vi "OTP - Main UI.vi"() -> ()   [LabVIEW 2020]
uses:
  Tab control.ctl
panel:
  in  "Back":bool
  in  "Tab Control":T1=enum."Source data"
  in  "Equipment":enum16{"VNA", "LCR"}(ring) caption="Equipment used for the beam data"
  in  "Measurement file (csv)":path
  in  "Frequency (MHz)":dbl=837.0
  in  "Package number":string="08"
  out "Cmax (fF)":dbl caption="Cmax measured (fF)"
  out "Cmin (fF)":dbl caption="Cmin measured (fF)"
  in  "Specification":T2={"Cmin (fF)"=500.0, "Cmin tolerance (%)"=10.0, "Cmax (fF)"=3460.0, "Cmax tolerance (%)"=1.38, "States"=32}
  out "Register 2 & 3 (hex) 2":string[][](array[string]) caption="Registers 2 & 3 (hex) to be considered"
  out "Register 2 & 3 (hex)":u8[][](array[numeric]) caption="Proposal for programming Register 2 & 3 (dec)"
  out "Results":dbl[][](array[numeric]) caption="Spec, Emulated, Error"
  in  "Save header":bool=TRUE
  in  "Write to device":bool=TRUE
  in  "Delay":u32=200 caption="Delay between writes (ms)"
  in  "PIC COM-port":refnum<visa-resource-name>
  in  "DUT info to write":T3={"Serial Number"=11, "Specification ID"="1A", "Variant"="W0", "Package"="22"}
  out "Status":string
  in  "Stop":bool
  in  "Forward":bool
  out "error out":errorcluster
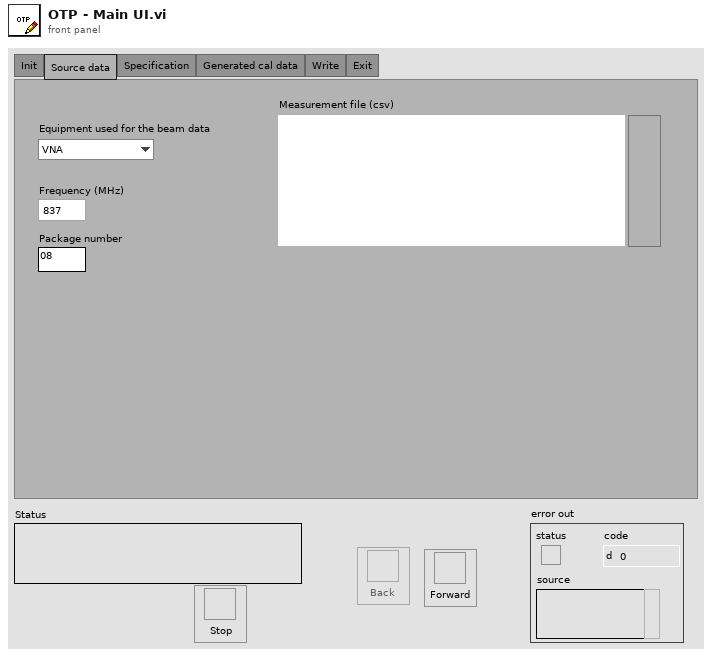
[diagram p1: front panel]
types:
  T1 = typedef "Tab control.ctl" = enum32{"Init", "Source data", "Specification", "Generated cal data", "Write", "Exit"}
  T2 = cluster{"Cmin (fF)":dbl, "Cmin tolerance (%)":dbl, "Cmax (fF)":dbl, "Cmax tolerance (%)":dbl, "States":i32}
  T3 = cluster{"Serial Number":u16, "Specification ID":string, "Variant":string, "Package":string}
  T4 = cluster{"Specification":cluster{"Cmin (fF)":dbl, "Cmin tolerance (%)":dbl, "Cmax (fF)":dbl, "Cmax tolerance (%)":dbl, "States":i32}, "Register 2 & 3 (hex)":string[][], "dCap (fF)":dbl[], "Cmin (fF)":dbl, "Cmax (fF)":dbl}
  T5 = cluster{"Package number":string, "Frequency (MHz)":dbl, "Measurement file (csv)":path, "Equipment":enum16{"VNA", "LCR"}}
  T6 = enum8{"Enabled", "Disabled", "Disabled and Grayed Out"}
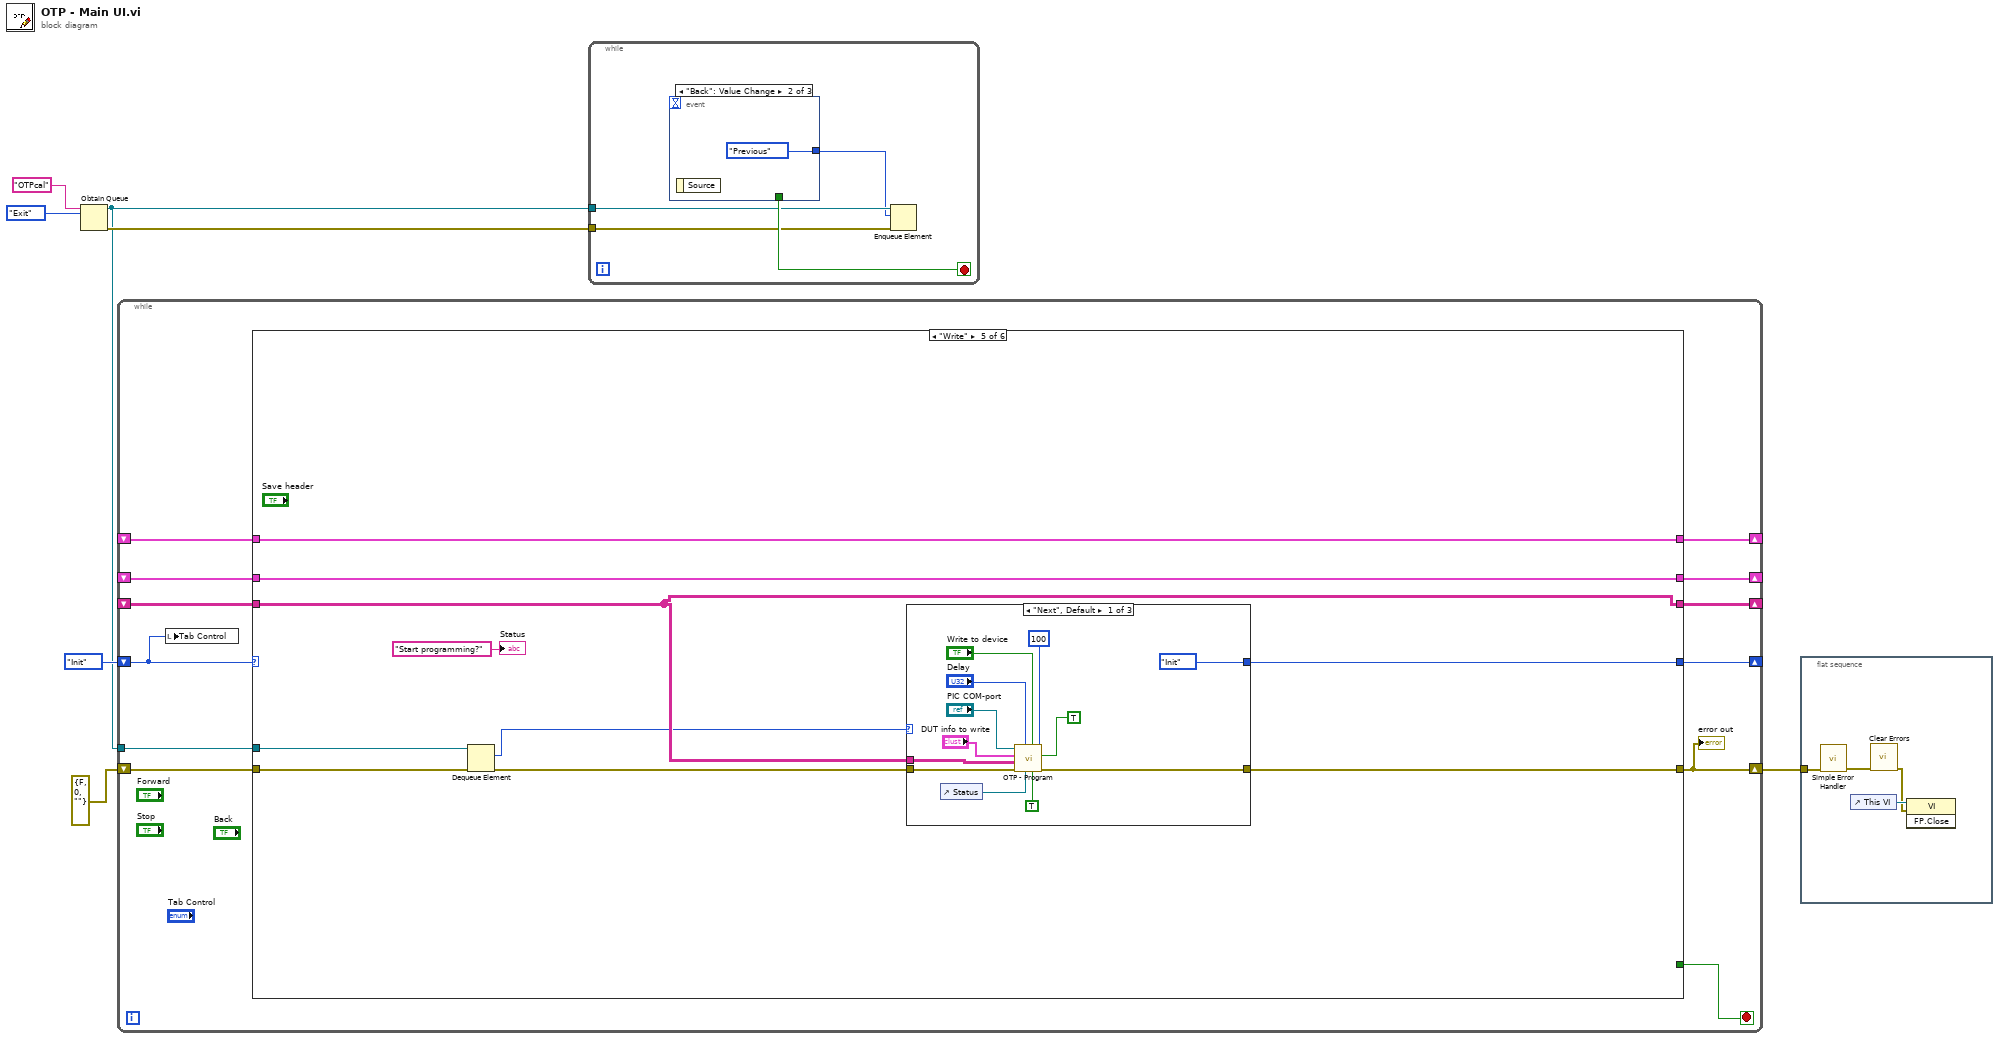
[diagram p0: block diagram]
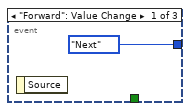
[diagram p2: hidden frame]
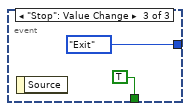
[diagram p3: hidden frame]
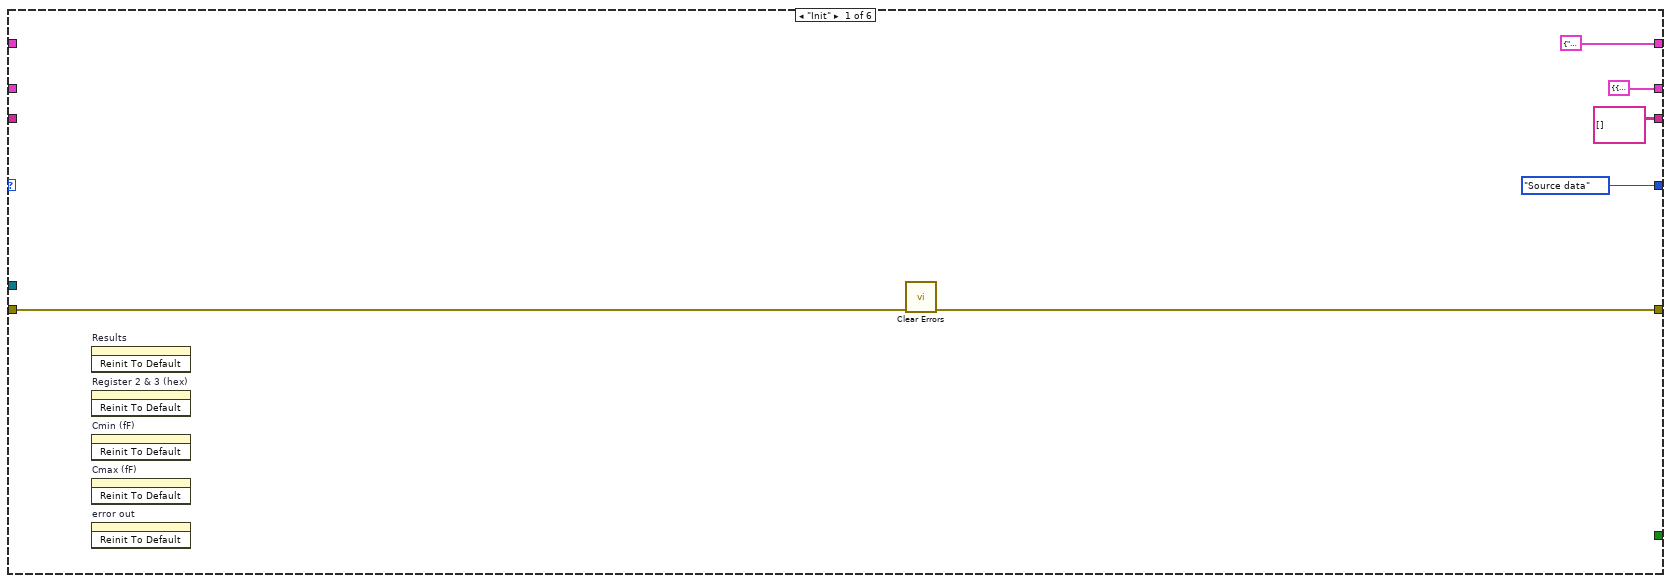
[diagram p4: hidden frame]
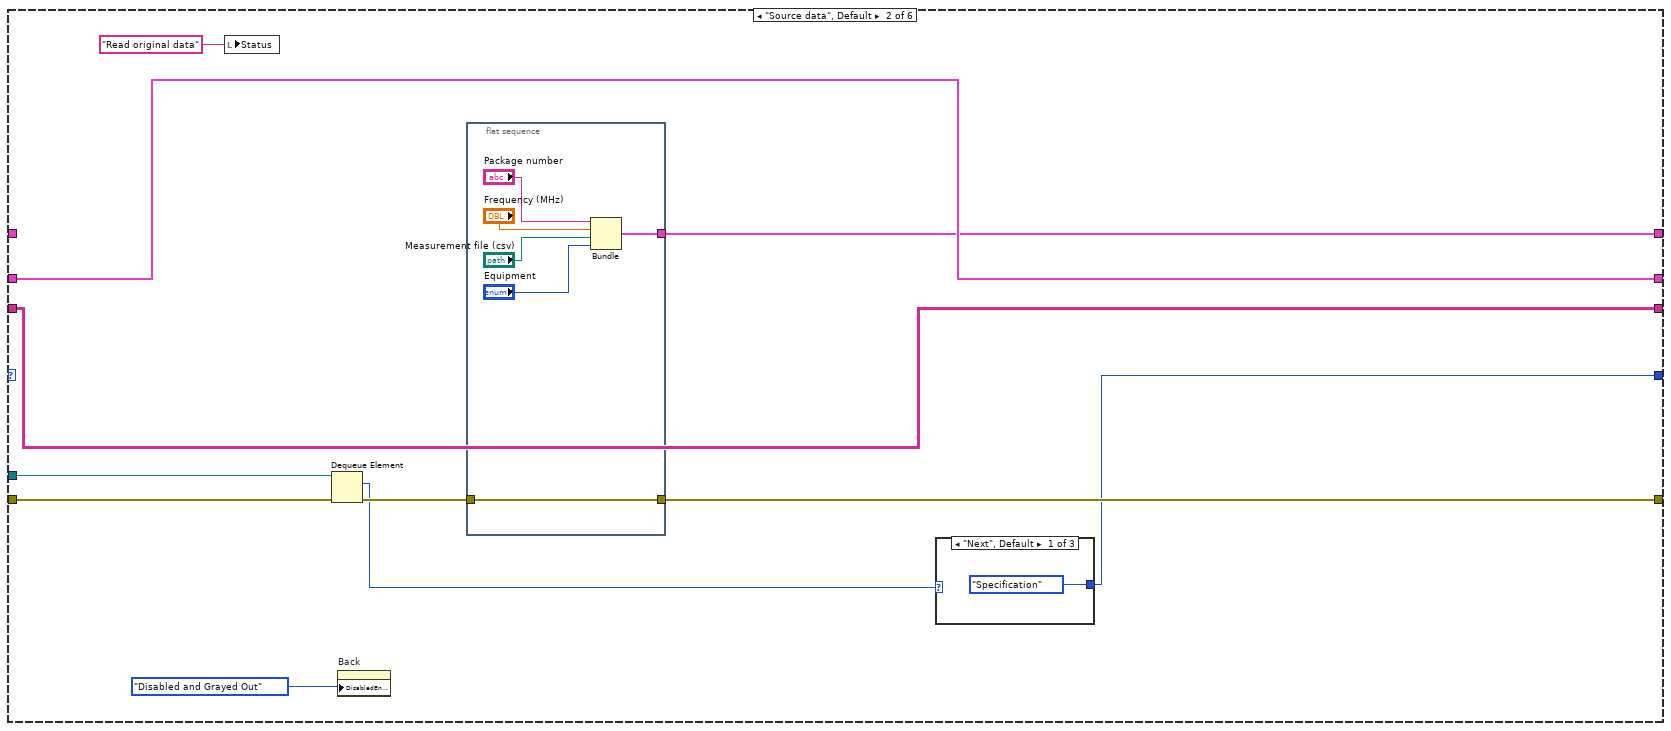
[diagram p5: hidden frame]
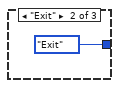
[diagram p6: hidden frame]
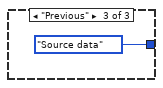
[diagram p7: hidden frame]
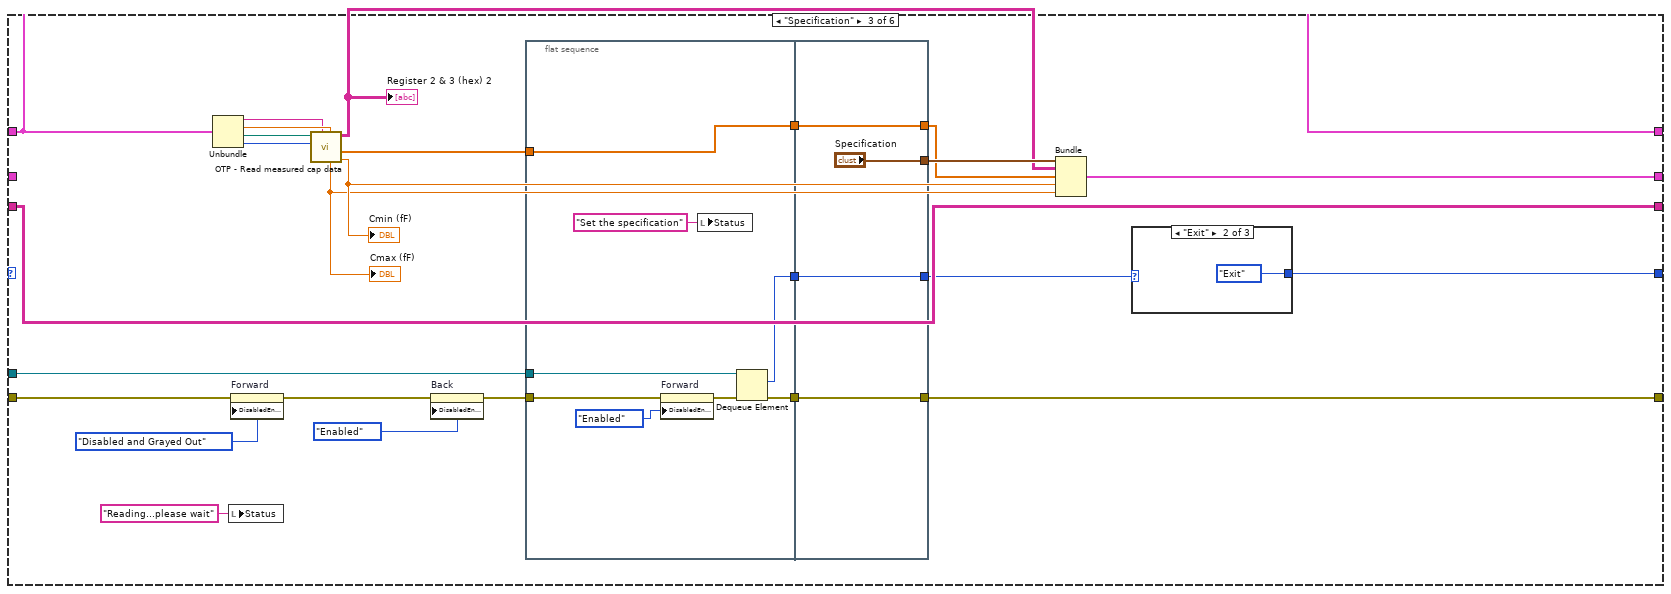
[diagram p8: hidden frame]
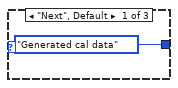
[diagram p9: hidden frame]
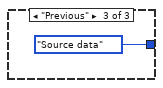
[diagram p10: hidden frame]
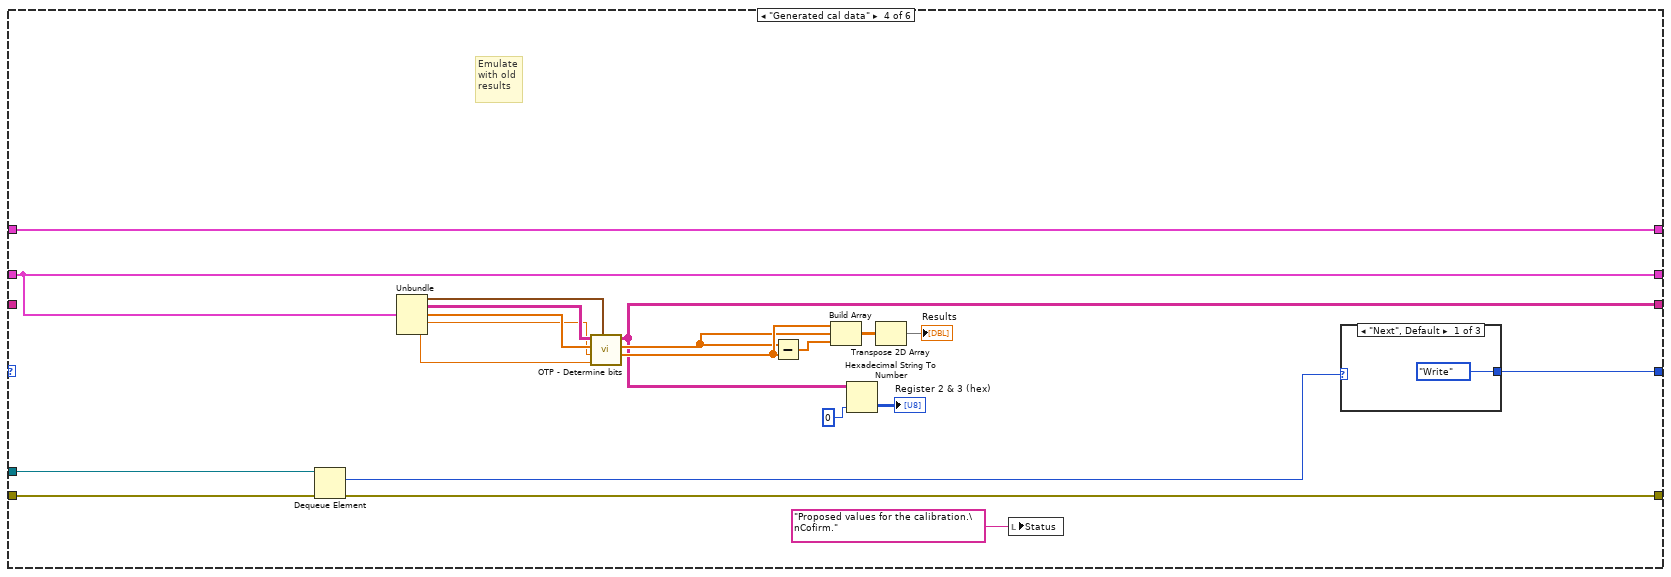
[diagram p11: hidden frame]
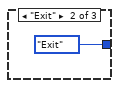
[diagram p12: hidden frame]
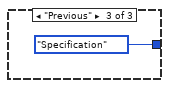
[diagram p13: hidden frame]
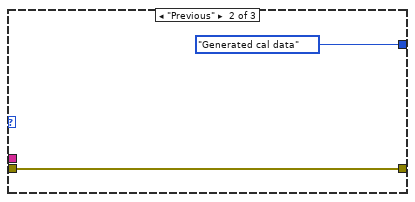
[diagram p14: hidden frame]
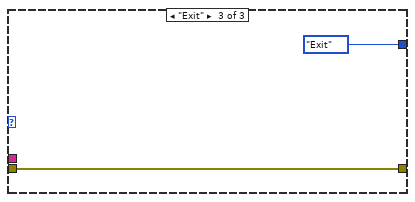
[diagram p15: hidden frame]
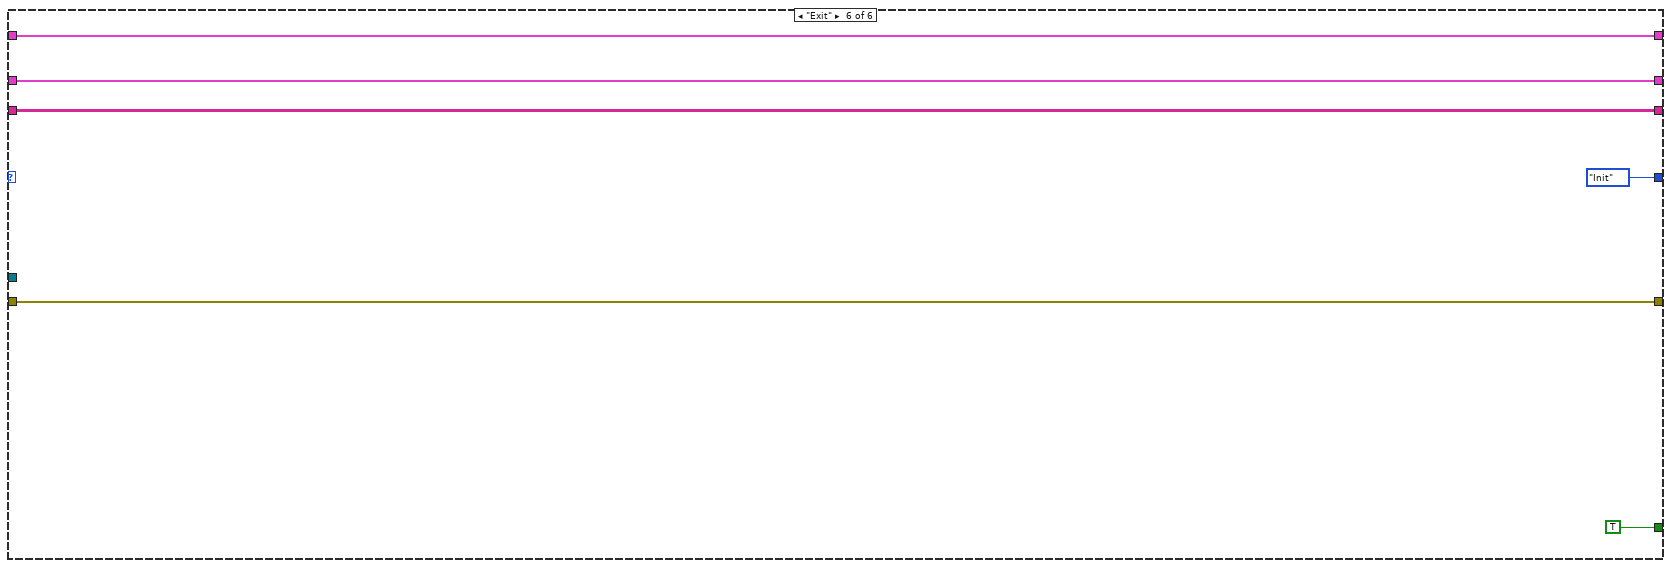
[diagram p16: hidden frame]
diagram:
  n1 = Obtain Queue(name (unnamed)="OTPcal", element data type=enum16{"Next", "Previous", "Exit"}."Exit") -> (queue out=w1:refnum<queue>, error out=w2:errorcluster)  [unwired: 3 in, 1 out]
  n2 = while {
    shift-right: [w18] -> _
    shift-left: Tab_control."Init" ("Tab Control") -> [w19]
    shift-right: [w10] -> _
    shift-left: _ -> [w16]
    shift-right: [w17] -> _
    shift-left: _ -> [w15]
    shift-right: [w14] -> _
    shift-left: _ -> [w13]
    shift-right: [w9] -> w6
    shift-left: errorcluster {"status"=FALSE, "code"=0, "source"=""} ("error out 2") -> [w12]
    tunnel: w1 -> [w8]
    stop <- w11 stop-if-true
    n3 = local write "Tab Control"(w19) -> ()
    n4 = case shown="\"Write\"" w19 {
      tunnel: [Tab_control."Source data" ("Tab Control") w27 w46 w88 w111 Tab_control."Init" ("Tab Control")] -> w18
      tunnel: [T5 {"Package number"="", "Frequency (MHz)"=0.0, "Measurement file (csv)"=path "", "Equipment"=enum."VNA"} w34 w56 w95 w117 w140] -> w10
      tunnel: [T4 {"Specification"={"Cmin (fF)"=0.0, "Cmin tolerance (%)"=0.0, "Cmax (fF)"=0.0, "Cmax tolerance (%)"=0.0, "States"=0}, "Register 2 & 3 (hex)"=[], "dCap (fF)"=[], "Cmin (fF)"=0.0, "Cmax (fF)"=0.0} w36 w61 w94 w118 w141] -> w17
      tunnel: w16 -> [_ _ w56 w95 w117 w140]
      tunnel: w15 -> [_ w36 _ w94 w118 w141]
      tunnel: [string[][] [] ("Register 2 & 3 (hex)") w35 w57 w96 w119 w142] -> w14
      tunnel: [w20 w30 w49 w90 w120 w138] -> w9
      tunnel: w13 -> [_ w35 w57 _ w119 w142]
      tunnel: w12 -> [w21 w32 w59 w91 w113 w138]
      tunnel: [_ _ _ _ _ TRUE] -> w11
      tunnel: w8 -> [_ w29 w50 w89 w115 _]
      frame "Init" {
        n5 = invoke on="Results" class="Arr (strict)" method="Reinit To Default"() -> ()  [unwired: 3 in, 3 out]
        n6 = invoke on="Register 2 & 3 (hex)" class="Arr (strict)" method="Reinit To Default"() -> ()  [unwired: 3 in, 3 out]
        n7 = invoke on="Cmin (fF)" class="DigNum (strict)" method="Reinit To Default"() -> ()  [unwired: 3 in, 3 out]
        n8 = invoke on="Cmax (fF)" class="DigNum (strict)" method="Reinit To Default"() -> ()  [unwired: 3 in, 3 out]
        n9 = invoke on="error out" class="Clust (strict)" method="Reinit To Default"() -> ()  [unwired: 3 in, 3 out]
        n10 = call <vilib>:"Clear Errors.vi"("error in (no error)"=w21) -> ("error out"=w20:errorcluster)  [unwired: 5 in, 1 out]
      }
      frame "Source data", Default {
        n11 = local write "Status"("Read original data" ("String")) -> ()
        n12 = Dequeue Element(queue=w29, error in (no error)=w32) -> (element=w28:enum16{"Next", "Previous", "Exit"}, error out=w31:errorcluster)  [unwired: 1 in, 2 out]
        n13 = property on="Back" class="Bool"("DisabledEnum"=T6."Disabled and Grayed Out" ("Disabled")) -> ()  [unwired: 2 in, 2 out]
        n14 = flat-sequence {
          tunnel: [w45] -> w34
          tunnel: [w40] -> w30
          tunnel: w31 -> [w40]
          frame #0 {
            n15 = Bundle("Package number"="Package number", "Frequency (MHz)"="Frequency (MHz)", "Measurement file (csv)"="Measurement file (csv)", "Equipment"="Equipment") -> (w45:T5)  [unwired: 1 in]
          }
        }
        n16 = case shown="\"Next\", Default" w28 {
          tunnel: [Tab_control."Specification" ("Tab Control") Tab_control."Exit" ("Tab Control") Tab_control."Source data" ("Tab Control")] -> w27
          frame "Next", Default {
          }
          frame "Exit" {
          }
          frame "Previous" {
          }
        }
      }
      frame "Specification" {
        n17 = Unbundle(w56) -> ("Package number"=w64:string, "Frequency (MHz)"=w65:dbl, "Measurement file (csv)"=w66:path, "Equipment"=w67:enum16{"VNA", "LCR"})
        n18 = local write "Status"("Reading...please wait" ("String")) -> ()
        n19 = property on="Forward" class="Bool"(error in=w59, "DisabledEnum"=T6."Disabled and Grayed Out" ("Disabled")) -> (error out=w58:errorcluster)  [unwired: 1 in, 1 out]
        n20 = call "OTP - Read measured cap data.vi"("Frequency (MHz)"=w65, "Package number"=w64, "Equipment"=w67, "file (use dialog)"=w66) -> ("Cmin (fF)"=w71:dbl, "dCap (fF)"=w53:dbl[], "Register 2 & 3 (hex)"=w68:string[][], "Cmax (fF)"=w69:dbl)  [unwired: 3 in, 1 out]
        "Cmin (fF)" <- w71
        "Cmax (fF)" <- w69
        "Register 2 & 3 (hex) 2" <- w68
        n21 = property on="Back" class="Bool"(error in=w58, "DisabledEnum"=T6."Enabled" ("Disabled")) -> (error out=w51:errorcluster)  [unwired: 1 in, 1 out]
        n22 = flat-sequence {
          tunnel: [w77] -> w55
          tunnel: [w80] -> w54
          tunnel: w53 -> [w80]
          tunnel: w51 -> [w79]
          tunnel: w50 -> [w78]
          tunnel: [w76] -> w48
          tunnel: [w86] -> w47
          tunnel: ["Specification"] -> w70
          tunnel: w55 -> [w86]
          tunnel: [w84] -> w52
          tunnel: w54 -> [w84]
          tunnel: [w83] -> w49
          tunnel: w48 -> [w83]
          frame #0 {
            n23 = property on="Forward" class="Bool"(error in=w79, "DisabledEnum"=T6."Enabled" ("Disabled")) -> (error out=w82:errorcluster)  [unwired: 1 in, 1 out]
            n24 = local write "Status"("Set the specification" ("String")) -> ()
            n25 = Dequeue Element(queue=w78, error in (no error)=w82) -> (element=w77:enum16{"Next", "Previous", "Exit"}, error out=w76:errorcluster)  [unwired: 1 in, 2 out]
          }
          frame #1 {
          }
        }
        n26 = Bundle("Specification"=w70, "Register 2 & 3 (hex)"=w68, "dCap (fF)"=w52, "Cmin (fF)"=w71, "Cmax (fF)"=w69) -> (w61:T4)  [unwired: 1 in]
        n27 = case shown="\"Exit\"" w47 {
          tunnel: [Tab_control."Generated cal data" ("Tab Control") Tab_control."Exit" ("Tab Control") Tab_control."Source data" ("Tab Control")] -> w46
          frame "Next", Default {
          }
          frame "Exit" {
          }
          frame "Previous" {
          }
        }
      }
      frame "Generated cal data" {
        # "Emulate\nwith old\nresults"
        n28 = Dequeue Element(queue=w89, error in (no error)=w91) -> (element=w87:enum16{"Next", "Previous", "Exit"}, error out=w90:errorcluster)  [unwired: 1 in, 2 out]
        n29 = Unbundle(w94) -> ("Specification"=w101:T2, "Register 2 & 3 (hex)"=w100:string[][], "dCap (fF)"=w99:dbl[], "Cmin (fF)"=w98:dbl, "Cmax (fF)"=w97:dbl)
        n30 = call "OTP - Determine bits.vi"("Specification"=w101, "Cmax measured (fF)"=w97, "Cmin measured (fF)"=w98, "dCap (fF)"=w99, "Register 2 & 3 (hex)"=w100) -> ("Target values (fF)"=w103:dbl[], "Measured values (fF)"=w102:dbl[], "Register 2 & 3 (hex)"=w96:string[][])  [unwired: 4 in]
        n31 = Subtract(x=w102, y=w103) -> (x-y=w104:dbl[])
        n32 = Build Array(w103, w102, w104) -> (w107:dbl[][])
        n33 = Hexadecimal String To Number(string=w96, default (0uL)=u8 0 ("milliseconds to wait")) -> (number=→"Register 2 & 3 (hex)":u8[][])  [unwired: 1 in, 1 out]
        n34 = Transpose 2D Array(2D array=w107) -> (transposed array=→"Results":dbl[][])
        n35 = local write "Status"("Proposed values for the calibration.\nCofirm." ("String")) -> ()
        n36 = case shown="\"Next\", Default" w87 {
          tunnel: [Tab_control."Write" ("Tab Control") Tab_control."Exit" ("Tab Control") Tab_control."Specification" ("Tab Control")] -> w88
          frame "Next", Default {
          }
          frame "Exit" {
          }
          frame "Previous" {
          }
        }
      }
      frame "Write" {
        n37 = Dequeue Element(queue=w115, error in (no error)=w113) -> (element=w112:enum16{"Next", "Previous", "Exit"}, error out=w114:errorcluster)  [unwired: 1 in, 2 out]
        n38 = case shown="\"Next\", Default" w112 {
          tunnel: w119 -> [w132 _ _]
          tunnel: [w124 w133 w135] -> w120
          tunnel: w114 -> [w123 w133 w135]
          tunnel: [Tab_control."Init" ("Tab Control") Tab_control."Generated cal data" ("Tab Control") Tab_control."Exit" ("Tab Control")] -> w111
          frame "Next", Default {
            n39 = control-ref of="Status"() -> (w125:refnum<vi>)
            n40 = call "OTP - Program.vi"("Save header"=TRUE, "Max number of retries"=100, "Read back the values written"=TRUE, "Write to device"="Write to device", "Str Refnum"=w125, "Delay"="Delay", "Error In"=w123, "OTP-cal registers 2 & 3 (hex)"=w132, "DUT info to write"="DUT info to write", "VISA resource name"="PIC COM-port") -> ("error out"=w124:errorcluster)  [unwired: 1 in]
          }
          frame "Previous" {
          }
          frame "Exit" {
          }
        }
        "Status" <- "Start programming?" ("String")
      }
      frame "Exit" {
      }
    }
    "error out" <- w9
  }
  n41 = while {
    tunnel: w1 -> [w145]
    tunnel: w2 -> [w144]
    stop <- w146 stop-if-true
    n42 = event shown="[1] \"Back\": Value Change" {
      selector: _ -> [_ _ _]
      dyn-events: _ -> [_ _ _]
      timeout: _ -> [_ _ _]
      tunnel: [enum16{"Next", "Previous", "Exit"}."Next" enum16{"Next", "Previous", "Exit"}."Previous" enum16{"Next", "Previous", "Exit"}."Exit"] -> w143
      tunnel: [_ _ TRUE] -> w146
      event "Forward": Value Change {
        n43 = event-data() -> ()  [unwired: 1 in, 1 out]
      }
      event "Back": Value Change {
        n44 = event-data() -> ()  [unwired: 1 in, 1 out]
      }
      event "Stop": Value Change {
        n45 = event-data() -> ()  [unwired: 1 in, 1 out]
      }
    }
    n46 = Enqueue Element(queue=w145, element=w143, error in (no error)=w144) -> ()  [unwired: 1 in, 3 out]
  }
  n47 = flat-sequence {
    tunnel: w6 -> [w153]
    frame #0 {
      n48 = call <vilib>:"Simple Error Handler.vi"("error in (no error)"=w153) -> ("error out"=w152:errorcluster)  [unwired: 4 in, 4 out]
      n49 = control-ref of="This VI"() -> (w154:refnum<vi>)
      n50 = call <vilib>:"Clear Errors.vi"("error in (no error)"=w152) -> ("error out"=w151:errorcluster)  [unwired: 5 in, 1 out]
      n51 = invoke class="VI" method="FP.Close"(reference=w154, error in=w151) -> ()  [unwired: 1 in, 3 out]
    }
  }
